vi "TSM DMM Initialize Sessions.vi"(0 "TSM context":T1) -> (15 "error out":errorcluster)   [LabVIEW 2020]
doc: "Use this VI to initialize sessions for all NI-DMM instruments in the pin map associated with the test program."
uses:
  <vilib>/NI_TestStand_SemiconductorModule/NI_TestStand_Semiconductor_Module.lvlibp/PinMap/General/SemiconductorModuleContext.ctl
  <vilib>/NI_TestStand_SemiconductorModule/NI_TestStand_Semiconductor_Module.lvlibp
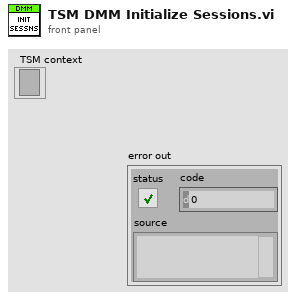
[diagram p1: front panel]
types:
  T1 = typedef "NI_TestStand_Semiconductor_Module.lvlibp/SemiconductorModuleContext.ctl" = refnum<k7>
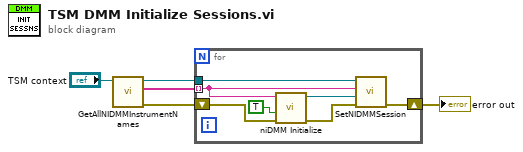
[diagram p0: block diagram]
diagram:
  n1 = call <vilib>:"GetAllNIDMMInstrumentNames.vi"("Semiconductor Module Context"="TSM context") -> ("error out"=w2:errorcluster, "Instrument Names"=w5:string[], "Semiconductor Module Context Out"=w4:T1)  [unwired: 8 in]
  n2 = for {
    tunnel: w5 -> [w10] mode=indexing
    tunnel: w4 -> [w7]
    shift-right: [w8] -> w1
    shift-left: w2 -> [w12]
    n3 = call <instrlib>:"niDMM Initialize.vi"("error in (no error)"=w12, "Reset"=TRUE, "Instrument Descriptor"=w10) -> ("error out"=w11:errorcluster, "instrument handle out"=w9:refnum<k15>)  [unwired: 7 in]
    n4 = call <vilib>:"SetNIDMMSession.vi"("error in (no error)"=w11, "Instrument Session"=w9, "Instrument Name"=w10, "Semiconductor Module Context"=w7) -> ("error out"=w8:errorcluster)  [unwired: 6 in, 1 out]
  }
  "error out" <- w1
